vi "LabVIEW-Interface.vi"() -> ()   [LabVIEW 2016]
panel:
  in  "Tab Control":enum32{"Maestro", "Esclavo"}(tab)
  in  "LED 2":bool
  in  "LED 1":bool
  in  "LED 4":bool
  in  "LED 3":bool
  out "DIP 1":bool
  out "DIP 2":bool
  out "DIP 3":bool
  out "DIP 4":bool
  in  "stop 2":bool
  in  "Serial Port 2":refnum<visa-resource-name>="COM13"
  out "DIP 5":bool
  out "DIP 6":bool
  out "DIP 7":bool
  out "DIP 8":bool
  in  "stop":bool
  in  "LED 7":bool
  in  "LED 8":bool
  in  "LED 5":bool
  in  "LED 6":bool
  in  "PWM":i32
  out "Temperatura 2":dbl(slide) scale=15.0..30.0
  out "Temperatura":dbl
  in  "Serial Port":refnum<visa-resource-name>="COM13"
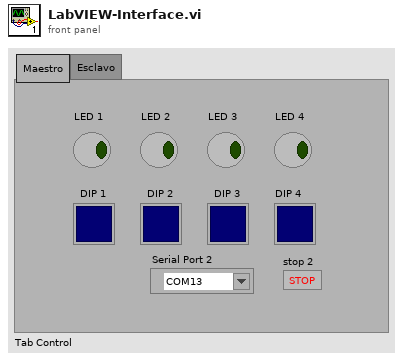
[diagram p1: front panel]
types:
  T1 = cluster{bool, bool, bool, bool, "LED 5":bool, "LED 6":bool, "LED 7":bool, "LED 8":bool}
  T2 = cluster{"Boolean array[0]":bool, "Boolean array[1]":bool, "Boolean array[2]":bool, "Boolean array[3]":bool, "Boolean array[4]":bool, "Boolean array[5]":bool, "Boolean array[6]":bool, "Boolean array[7]":bool, "Boolean array[8]":bool}
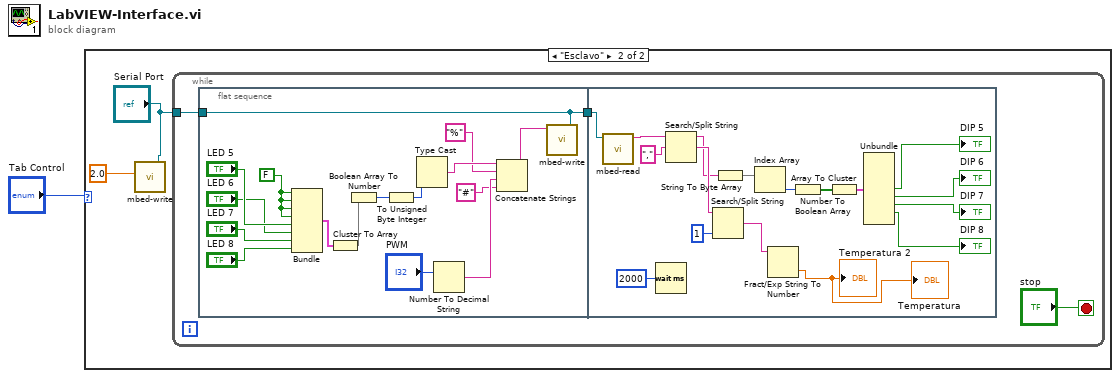
[diagram p0: block diagram]
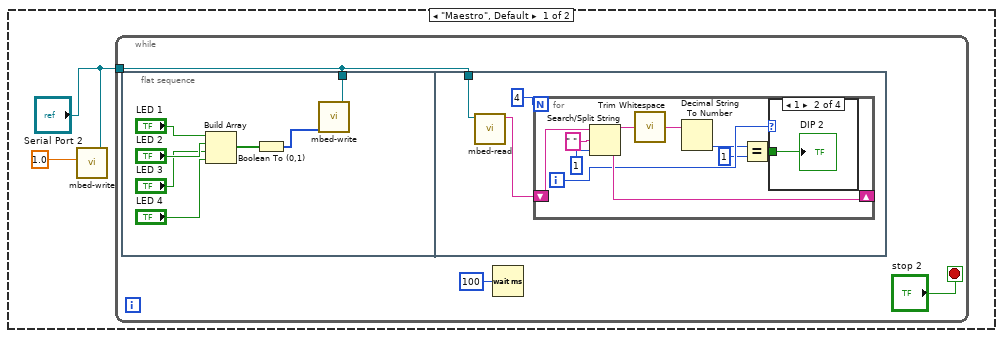
[diagram p2: hidden frame]
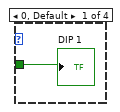
[diagram p3: hidden frame]
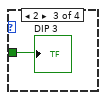
[diagram p4: hidden frame]
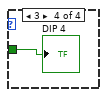
[diagram p5: hidden frame]
diagram:
  n1 = case shown="\"Esclavo\"" "Tab Control" {
    frame "Maestro", Default {
      n2 = call <vilib>:"mbed-write.vi"("Serial Port"="Serial Port 2", "Number"=1.0) -> ()  [unwired: 5 in, 1 out]
      n3 = while {
        tunnel: "Serial Port 2" -> [w4]
        stop <- "stop 2" stop-if-true
        n4 = flat-sequence {
          tunnel: w4 -> [w13]
          tunnel: w4 -> [w16]
          frame #0 {
            n5 = Build Array("LED 1", "LED 2", "LED 3", "LED 4") -> (w8:bool[])
            n6 = Boolean To (0,1)(Boolean=w8) -> (0, 1=w7:i16[])
            n7 = call <vilib>:"mbed-write.vi"("Serial Port"=w13, "Array of Numbers"=w7) -> ()  [unwired: 5 in, 1 out]
          }
          frame #1 {
            n8 = call <vilib>:"mbed-read.vi"("Serial Port"=w16) -> ("Line String"=w15:string)  [unwired: 3 in, 3 out]
            n9 = for {
              N: 4 -> [_]
              shift-right: [w24] -> _
              shift-left: w15 -> [w26]
              i -> [w20]
              n10 = Search/Split String(string=w26, search string/char (-)=" ", offset (0)=1) -> (substring before match=w22:string, match + rest of string=w24:string)  [unwired: 1 out]
              n11 = call <vilib>:"Trim Whitespace.vi"("string"=w22) -> ("trimmed string"=w21:string)  [unwired: 1 in]
              n12 = Decimal String To Number(string=w21) -> (number=w19:i32)  [unwired: 2 in, 1 out]
              n13 = Equal?(x=w19, y=1) -> (x = y?=w17:bool)
              n14 = case shown="1" w20 {
                tunnel: w17 -> [w27 w28 w29 w30]
                frame 0, Default {
                  "DIP 1" <- w27
                }
                frame 1 {
                  "DIP 2" <- w28
                }
                frame 2 {
                  "DIP 3" <- w29
                }
                frame 3 {
                  "DIP 4" <- w30
                }
              }
            }
          }
        }
        n15 = Wait (ms)(milliseconds to wait=u32 100) -> ()  [unwired: 1 out]
      }
    }
    frame "Esclavo" {
      n16 = call <vilib>:"mbed-write.vi"("Serial Port"="Serial Port", "Number"=2.0) -> ()  [unwired: 5 in, 1 out]
      n17 = while {
        tunnel: "Serial Port" -> [w34]
        stop <- "stop" stop-if-true
        n18 = flat-sequence {
          tunnel: w34 -> [w36]
          tunnel: [w36] -> w33
          tunnel: w33 -> [w53]
          frame #0 {
            w47 = FALSE
            n19 = Bundle(w47, w47, w47, w47, "LED 5"="LED 5", "LED 6"="LED 6", "LED 7"="LED 7", "LED 8"="LED 8") -> (w48:T1)  [unwired: 1 in]
            n20 = Cluster To Array(cluster=w48) -> (array=w51:bool[])
            n21 = Boolean Array To Number(Boolean array=w51) -> (number=w50:u32)
            n22 = To Unsigned Byte Integer(number=w50) -> (unsigned 8bit integer=w49:u8)
            n23 = Type Cast(x=w49) -> (*(type *) &x=w41:string)  [unwired: 1 in]
            n24 = Number To Decimal String(number="PWM") -> (decimal integer string=w39:string)  [unwired: 1 in]
            n25 = Concatenate Strings(w41, "%", w39, "#") -> (w37:string)
            n26 = call <vilib>:"mbed-write.vi"("Serial Port"=w36, "Line String"=w37) -> ()  [unwired: 5 in, 1 out]
          }
          frame #1 {
            n27 = call <vilib>:"mbed-read.vi"("Serial Port"=w53) -> ("Line String"=w63:string)  [unwired: 3 in, 3 out]
            n28 = Wait (ms)(milliseconds to wait=u32 2000) -> ()  [unwired: 1 out]
            n29 = Search/Split String(string=w63, search string/char (-)=",") -> (substring before match=w65:string, match + rest of string=w66:string)  [unwired: 1 in, 1 out]
            n30 = Search/Split String(string=w66, offset (0)=1) -> (match + rest of string=w68:string)  [unwired: 1 in, 2 out]
            n31 = String To Byte Array(string=w65) -> (unsigned byte array=w55:u8[])
            n32 = Index Array(array=w55) -> (element=w56:u8)  [unwired: 1 in]
            n33 = Fract/Exp String To Number(string=w68) -> (number=→"Temperatura 2" →"Temperatura":dbl)  [unwired: 3 in, 1 out]
            n34 = Number To Boolean Array(number=w56) -> (Boolean array=w57:bool[])
            n35 = Array To Cluster(array=w57) -> (cluster=w58:T2)
            n36 = Unbundle(w58) -> ("Boolean array[4]"=→"DIP 5":bool, "Boolean array[5]"=→"DIP 6":bool, "Boolean array[6]"=→"DIP 7":bool, "Boolean array[7]"=→"DIP 8":bool)  [unwired: 5 out]
          }
        }
      }
    }
  }
